vi "_Remote Get Turbo Status.vi"(0 "Update Info":bool, 1 "Update Temp":bool, 2 "Update Error":bool, 3 "Update Pumping":bool, 4 "Update Power":bool) -> (5 "Power / Current:":string[][](table)=[["Drive Power (W)", "0010031602=?105"], ["Drive Current (A)", "0010031002=?099"]], 6 "Turbo OK":bool, 7 "Pump Info:":string[][](table)=[["Hardware Version", "0010035402=?107"], ["Firmware Version", "0010031202=?101"], ["Operating Hours (Pump)", "0010031102=?100"], ["Operating Hours (Electronic Drive)", "0010031402=?103"]], 8 "Temperatures:":string[][](table)=[["Electronic Drive Temperature", "0010030402=?102"], ["Pump Temperature", "0010030502=?103"], ["Power Stage Temperature (°C)", "0010032402=?104"], ["Electronics Temperature (°C)", "0010032602=?106"], ["Upper Pump Temperature (°C)", "0010033002=?101"], ["Bearing Temperature (°C)", "0010034202=?104"], ["Motor Temperature (°C)", "0010034602=?108"]], 9 "Error History":string[][](table)=[["Current Error Code", "0010030302=?101", ""], ["Error Code History, 1", "0010036002=?104", ""], ["Error Code History, 2", "0010036102=?105", ""], ["Error Code History, 3", "0010036202=?106", ""], ["Error Code History, 4", "0010036302=?107", ""], ["Error Code History, 5", "0010036402=?108", ""], ["Error Code History, 6", "0010036502=?109", ""], ["Error Code History, 7", "0010036602=?110", ""], ["Error Code History, 8", "0010036702=?111", ""], ["Error Code History, 9", "0010036802=?112", ""], ["Error Code History, 10", "0010036902=?113", ""]], 10 "Pumping:":string[][](table)=[["Rotational Frequency (Hz)", "0010030902=?107"], ["Rotational Speed (rpm)", "0010039802=?115"]])   [LabVIEW 2012]
uses:
  Type/_Pump Parameter.ctl
  Configuration/_Global Configuration.vi
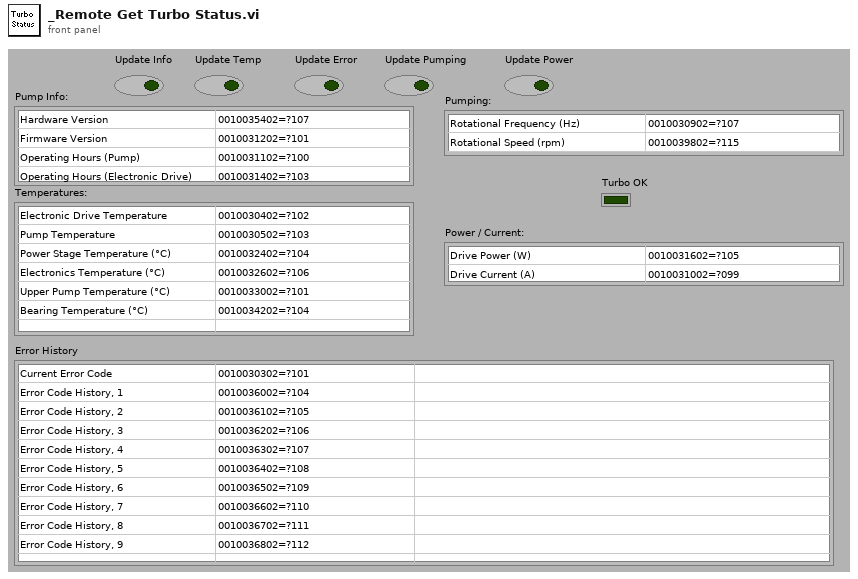
[diagram p1: front panel]
types:
  T1 = typedef "_Pump Parameter.ctl" = enum16{"Turn Pump Motor On", "Turn Pump Motor Off", "Read Pump Oil Deficiency", "Read Rotation Switch Point Attained", "Read Ele. Drive Over Temperature", "Read Pump Over Temperature", "Read Set Rotation Speed Attained", "Read Turbopump Accelerates", "Read Actual Rotation Speed in Hz", "Read Motor Current in A", "Read Operating Hours in h", "Read Motor Voltage in V", "Read Motor Power in W", "Set Rotation Speed Switchpoint in %", "Clear Error", "Read Error Code", "Read Bearing Temperature", "Read Hardware Version", "Read Firmware Version", "Read Operating Hours (Drive)", "Read Rotational Speed (rpm)", "Read Power Stage Temperature", "Read Electronics Temperature", "Read Upper Pump Temperature", "Read Motor Temperature", "Read Error Code History, 1", "Read Error Code History, 2", "Read Error Code History, 3", "Read Error Code History, 4", "Read Error Code History, 5", "Read Error Code History, 6", "Read Error Code History, 7", "Read Error Code History, 8", "Read Error Code History, 9", "Read Error Code History, 10"}
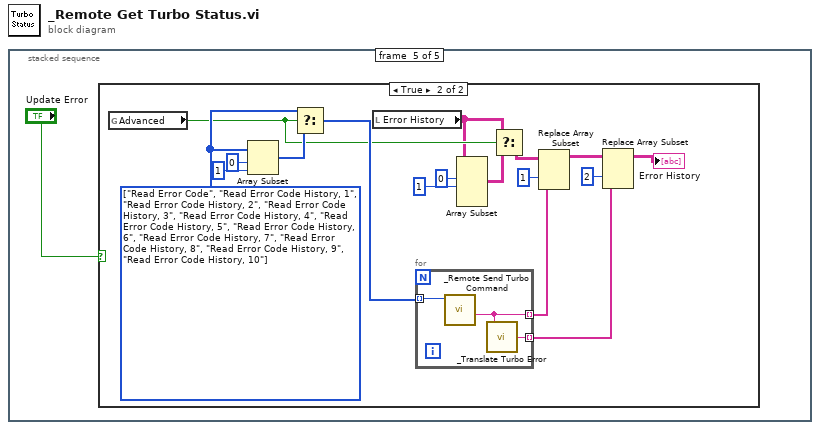
[diagram p0: block diagram]
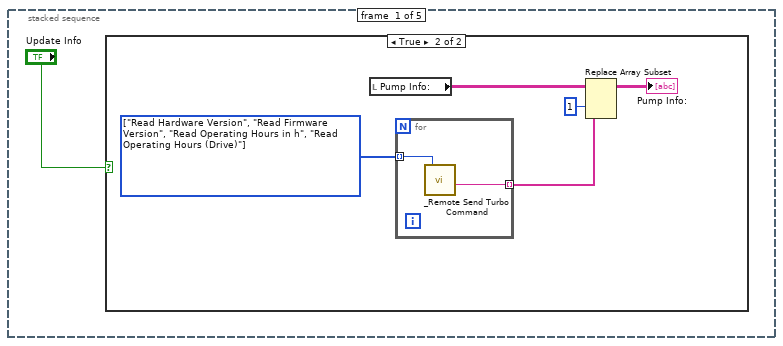
[diagram p2: hidden frame]
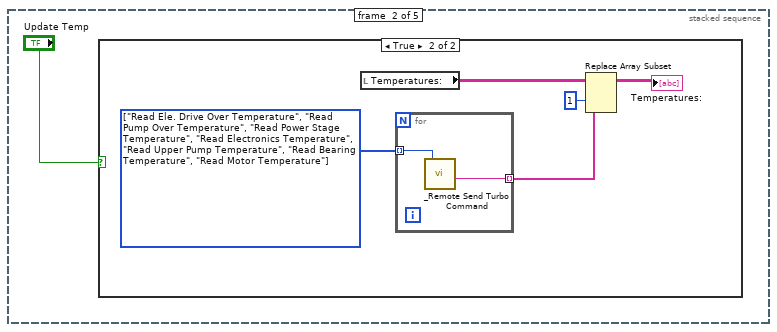
[diagram p4: hidden frame]
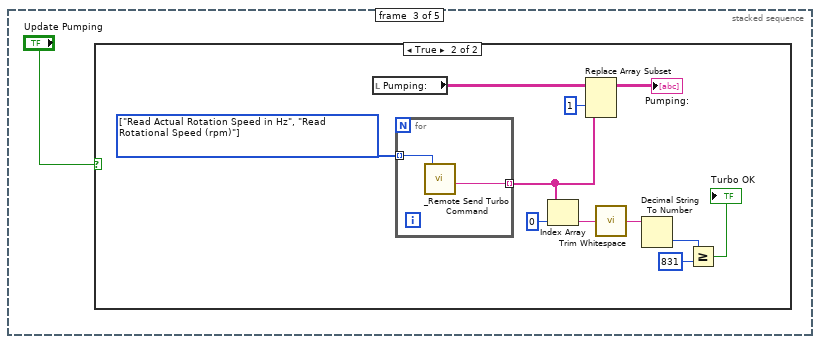
[diagram p6: hidden frame]
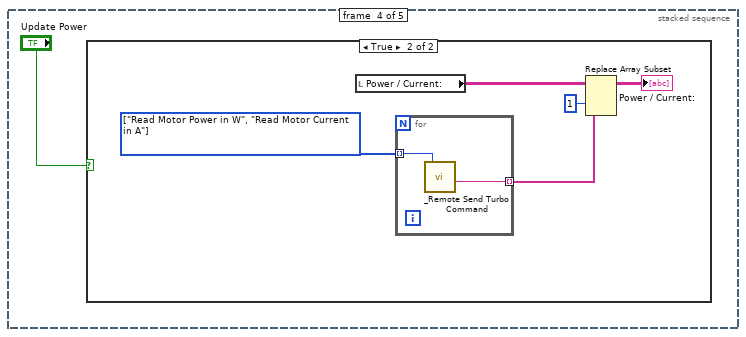
[diagram p8: hidden frame]
diagram:
  n1 = stacked-sequence {
    frame #0 {
      n2 = case shown="True" "Update Info" {
        frame False {
        }
        frame True {
          w6 = T1[] [enum."Read Hardware Version", enum."Read Firmware Version", enum."Read Operating Hours in h", enum."Read Operating Hours (Drive)"] items=["Turn Pump Motor On", "Turn Pump Motor Off", "Read Pump Oil Deficiency", "Read Rotation Switch Point Attained", "Read Ele. Drive Over Temperature", "Read Pump Over Temperature", "Read Set Rotation Speed Attained", "Read Turbopump Accelerates", "Read Actual Rotation Speed in Hz", "Read Motor Current in A", "Read Operating Hours in h", "Read Motor Voltage in V", "Read Motor Power in W", "Set Rotation Speed Switchpoint in %", "Clear Error", "Read Error Code", "Read Bearing Temperature", "Read Hardware Version", "Read Firmware Version", "Read Operating Hours (Drive)", "Read Rotational Speed (rpm)", "Read Power Stage Temperature", "Read Electronics Temperature", "Read Upper Pump Temperature", "Read Motor Temperature", "Read Error Code History, 1", "Read Error Code History, 2", "Read Error Code History, 3", "Read Error Code History, 4", "Read Error Code History, 5", "Read Error Code History, 6", "Read Error Code History, 7", "Read Error Code History, 8", "Read Error Code History, 9", "Read Error Code History, 10"]
          n3 = local read "Pump Info:"() -> (w5:string[][])
          n4 = for {
            tunnel: w6 -> [w8] mode=indexing
            tunnel: [w7] -> w4 mode=indexing
            n5 = call "_Remote Send Turbo Command.vi"("Pump Command"=w8) -> ("Data"=w7:string)  [unwired: 2 in, 4 out]
          }
          n6 = Replace Array Subset(array=w5, new element=w4, index (col)=1 ("disabled index (col)")) -> (→"Pump Info:":string[][])  [unwired: 1 in]
        }
      }
    }
    frame #1 {
      n7 = case shown="True" "Update Temp" {
        frame False {
        }
        frame True {
          w14 = T1[] [enum."Read Ele. Drive Over Temperature", enum."Read Pump Over Temperature", enum."Read Power Stage Temperature", enum."Read Electronics Temperature", enum."Read Upper Pump Temperature", enum."Read Bearing Temperature", enum."Read Motor Temperature"] items=["Turn Pump Motor On", "Turn Pump Motor Off", "Read Pump Oil Deficiency", "Read Rotation Switch Point Attained", "Read Ele. Drive Over Temperature", "Read Pump Over Temperature", "Read Set Rotation Speed Attained", "Read Turbopump Accelerates", "Read Actual Rotation Speed in Hz", "Read Motor Current in A", "Read Operating Hours in h", "Read Motor Voltage in V", "Read Motor Power in W", "Set Rotation Speed Switchpoint in %", "Clear Error", "Read Error Code", "Read Bearing Temperature", "Read Hardware Version", "Read Firmware Version", "Read Operating Hours (Drive)", "Read Rotational Speed (rpm)", "Read Power Stage Temperature", "Read Electronics Temperature", "Read Upper Pump Temperature", "Read Motor Temperature", "Read Error Code History, 1", "Read Error Code History, 2", "Read Error Code History, 3", "Read Error Code History, 4", "Read Error Code History, 5", "Read Error Code History, 6", "Read Error Code History, 7", "Read Error Code History, 8", "Read Error Code History, 9", "Read Error Code History, 10"]
          n8 = local read "Temperatures:"() -> (w13:string[][])
          n9 = for {
            tunnel: w14 -> [w16] mode=indexing
            tunnel: [w15] -> w12 mode=indexing
            n10 = call "_Remote Send Turbo Command.vi"("Pump Command"=w16) -> ("Data"=w15:string)  [unwired: 2 in, 4 out]
          }
          n11 = Replace Array Subset(array=w13, new element=w12, index (col)=1 ("disabled index (col)")) -> (→"Temperatures:":string[][])  [unwired: 1 in]
        }
      }
    }
    frame #2 {
      n12 = case shown="True" "Update Pumping" {
        frame False {
        }
        frame True {
          w28 = T1[] [enum."Read Actual Rotation Speed in Hz", enum."Read Rotational Speed (rpm)"] items=["Turn Pump Motor On", "Turn Pump Motor Off", "Read Pump Oil Deficiency", "Read Rotation Switch Point Attained", "Read Ele. Drive Over Temperature", "Read Pump Over Temperature", "Read Set Rotation Speed Attained", "Read Turbopump Accelerates", "Read Actual Rotation Speed in Hz", "Read Motor Current in A", "Read Operating Hours in h", "Read Motor Voltage in V", "Read Motor Power in W", "Set Rotation Speed Switchpoint in %", "Clear Error", "Read Error Code", "Read Bearing Temperature", "Read Hardware Version", "Read Firmware Version", "Read Operating Hours (Drive)", "Read Rotational Speed (rpm)", "Read Power Stage Temperature", "Read Electronics Temperature", "Read Upper Pump Temperature", "Read Motor Temperature", "Read Error Code History, 1", "Read Error Code History, 2", "Read Error Code History, 3", "Read Error Code History, 4", "Read Error Code History, 5", "Read Error Code History, 6", "Read Error Code History, 7", "Read Error Code History, 8", "Read Error Code History, 9", "Read Error Code History, 10"]
          n13 = local read "Pumping:"() -> (w27:string[][])
          n14 = for {
            tunnel: w28 -> [w30] mode=indexing
            tunnel: [w29] -> w21 mode=indexing
            n15 = call "_Remote Send Turbo Command.vi"("Pump Command"=w30) -> ("Data"=w29:string)  [unwired: 2 in, 4 out]
          }
          n16 = Index Array(array=w21, index=0) -> (element=w20:string)
          n17 = Replace Array Subset(array=w27, new element=w21, index (col)=1 ("disabled index (col)")) -> (→"Pumping:":string[][])  [unwired: 1 in]
          n18 = call <vilib>:"Trim Whitespace.vi"("string"=w20) -> ("trimmed string"=w22:string)  [unwired: 1 in]
          n19 = Decimal String To Number(string=w22) -> (number=w24:i32)  [unwired: 3 out]
          n20 = Greater Or Equal?(x=w24, y=831) -> (x >= y?=→"Turbo OK":bool)
        }
      }
    }
    frame #3 {
      n21 = case shown="True" "Update Power" {
        frame False {
        }
        frame True {
          w36 = T1[] [enum."Read Motor Power in W", enum."Read Motor Current in A"] items=["Turn Pump Motor On", "Turn Pump Motor Off", "Read Pump Oil Deficiency", "Read Rotation Switch Point Attained", "Read Ele. Drive Over Temperature", "Read Pump Over Temperature", "Read Set Rotation Speed Attained", "Read Turbopump Accelerates", "Read Actual Rotation Speed in Hz", "Read Motor Current in A", "Read Operating Hours in h", "Read Motor Voltage in V", "Read Motor Power in W", "Set Rotation Speed Switchpoint in %", "Clear Error", "Read Error Code", "Read Bearing Temperature", "Read Hardware Version", "Read Firmware Version", "Read Operating Hours (Drive)", "Read Rotational Speed (rpm)", "Read Power Stage Temperature", "Read Electronics Temperature", "Read Upper Pump Temperature", "Read Motor Temperature", "Read Error Code History, 1", "Read Error Code History, 2", "Read Error Code History, 3", "Read Error Code History, 4", "Read Error Code History, 5", "Read Error Code History, 6", "Read Error Code History, 7", "Read Error Code History, 8", "Read Error Code History, 9", "Read Error Code History, 10"]
          n22 = local read "Power / Current:"() -> (w35:string[][])
          n23 = for {
            tunnel: w36 -> [w38] mode=indexing
            tunnel: [w37] -> w34 mode=indexing
            n24 = call "_Remote Send Turbo Command.vi"("Pump Command"=w38) -> ("Data"=w37:string)  [unwired: 2 in, 4 out]
          }
          n25 = Replace Array Subset(array=w35, new element=w34, index (col)=1 ("disabled index (col)")) -> (→"Power / Current:":string[][])  [unwired: 1 in]
        }
      }
    }
    frame #4 {
      n26 = case shown="True" "Update Error" {
        frame False {
        }
        frame True {
          w47 = T1[] [enum."Read Error Code", enum."Read Error Code History, 1", enum."Read Error Code History, 2", enum."Read Error Code History, 3", enum."Read Error Code History, 4", enum."Read Error Code History, 5", enum."Read Error Code History, 6", enum."Read Error Code History, 7", enum."Read Error Code History, 8", enum."Read Error Code History, 9", enum."Read Error Code History, 10"] items=["Turn Pump Motor On", "Turn Pump Motor Off", "Read Pump Oil Deficiency", "Read Rotation Switch Point Attained", "Read Ele. Drive Over Temperature", "Read Pump Over Temperature", "Read Set Rotation Speed Attained", "Read Turbopump Accelerates", "Read Actual Rotation Speed in Hz", "Read Motor Current in A", "Read Operating Hours in h", "Read Motor Voltage in V", "Read Motor Power in W", "Set Rotation Speed Switchpoint in %", "Clear Error", "Read Error Code", "Read Bearing Temperature", "Read Hardware Version", "Read Firmware Version", "Read Operating Hours (Drive)", "Read Rotational Speed (rpm)", "Read Power Stage Temperature", "Read Electronics Temperature", "Read Upper Pump Temperature", "Read Motor Temperature", "Read Error Code History, 1", "Read Error Code History, 2", "Read Error Code History, 3", "Read Error Code History, 4", "Read Error Code History, 5", "Read Error Code History, 6", "Read Error Code History, 7", "Read Error Code History, 8", "Read Error Code History, 9", "Read Error Code History, 10"]
          n27 = global read "_Global Configuration.vi" "Advanced"() -> (w45:bool)
          n28 = Array Subset(array=w47, index=0, length=1) -> (w46:T1[])
          n29 = Select(t=w47, s=w45, f=w46) -> (s? t:f=w50:T1[])
          n30 = local read "Error History"() -> (w44:string[][])
          n31 = for {
            tunnel: w50 -> [w59] mode=indexing
            tunnel: [w57] -> w56 mode=indexing
            tunnel: [w58] -> w52 mode=indexing
            n32 = call "_Remote Send Turbo Command.vi"("Pump Command"=w59) -> ("Data"=w57:string)  [unwired: 2 in, 4 out]
            n33 = call "_Translate Turbo Error.vi"("Error Code"=w57) -> ("Translation"=w58:string)
          }
          n34 = Array Subset(array=w44, index (row)=0 ("index"), length (row)=1 ("length")) -> (w40:string[][])  [unwired: 2 in]
          n35 = Select(t=w44, s=w45, f=w40) -> (s? t:f=w43:string[][])
          n36 = Replace Array Subset(array=w43, new element=w56, index (col)=1 ("disabled index (col)")) -> (w53:string[][])  [unwired: 1 in]
          n37 = Replace Array Subset(array=w53, new element=w52, index (col)=2 ("disabled index (col)")) -> (→"Error History":string[][])  [unwired: 1 in]
        }
      }
    }
  }
